vi "Turn All Tubes ON-OFF.vi"(8 "Activate: 1\nDeactivate: 0":bool, 9 "Pins In":refnum<k21>[](array[refnum]), 10 "First Tube #":i32, 11 "Last Tube #":i32) -> (3 "Pins Out":refnum<k21>[](array[refnum]))   [LabVIEW 2020]
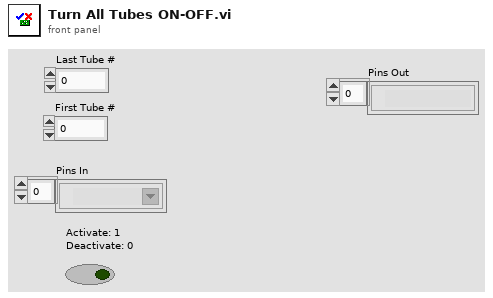
[diagram p1: front panel]
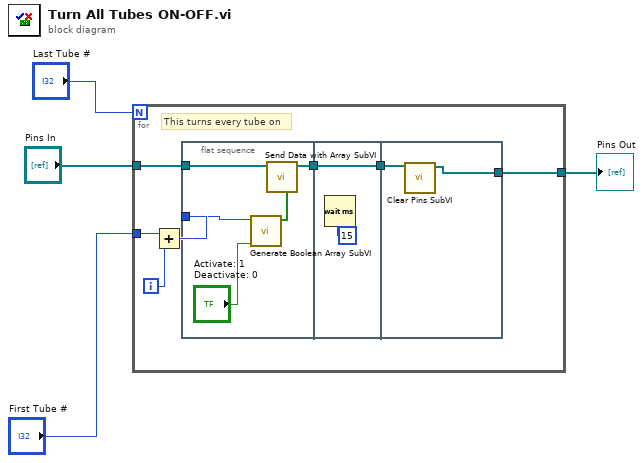
[diagram p0: block diagram]
diagram:
  n1 = for {
    N: "Last Tube #" -> [_]
    tunnel: "First Tube #" -> [w9]
    tunnel: "Pins In" -> [w8]
    tunnel: [w5] -> w2
    i -> [w10]
    # "This turns every tube on"
    n2 = Add(x=w9, y=w10) -> (x+y=w11:i32)
    n3 = flat-sequence {
      tunnel: w11 -> [w15]
      tunnel: w8 -> [w14]
      tunnel: [w13] -> w6
      tunnel: [w17] -> w7
      tunnel: w6 -> [w17]
      tunnel: w7 -> [w20]
      tunnel: [w19] -> w5
      frame #0 {
        n4 = call "Generate Boolean Array SubVI.vi"("Activate: 1\nDeactivate: 0"="Activate: 1\nDeactivate: 0", "Tube"=w15) -> ("Boolean array"=w16:bool[])  [unwired: 9 in]
        n5 = call "Send Data with Array SubVI.vi"("Pins In"=w14, "Data"=w16) -> ("Pins Out"=w13:refnum<k21>[])  [unwired: 7 in]
      }
      frame #1 {
        n6 = Wait (ms)(milliseconds to wait=u32 15) -> ()  [unwired: 1 out]
      }
      frame #2 {
        n7 = call "Clear Pins SubVI.vi"("Pins In"=w20) -> ("Pins Out"=w19:refnum<k21>[])  [unwired: 10 in]
      }
    }
  }
  "Pins Out" <- w2
